vi "PH_PILS.vis ResetEOKnob.vi"(0 "i ref in":refnum<vi>, 5 "error IO":errorcluster) -> (14 "i ref out":refnum<vi>, 19 "error out":errorcluster)   [LabVIEW 2014, in "PH_PILS.lvlib"]
uses:
  PH_PILS.lvlib
  PH_Basics/PH_SystemInformation/PH_SystemInformation.lvlib
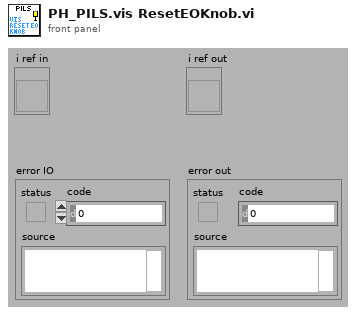
[diagram p1: front panel]
types:
  T1 = typedef "PH_PILS.lvlib/PH_PILS.i attribute.ctl" = cluster{"Boolean":cluster{"GUI Ref":refnum<vi>, "Status":i32}[], "GUI Refs Exp. Shutters":cluster{"1":refnum<vi>, "2":refnum<vi>, "3":refnum<vi>, "4":refnum<vi>}, "Tristate2Run GUI Refs":refnum<vi>[], "EO-Likes":cluster{"GUI Ref":refnum<vi>, "Status":i32}[], "Operation Mode":cluster{"Operation Mode":T2, "GUI":cluster{"Ref State":refnum<vi>, "Ref":refnum<vi>}, "Servicemode":cluster{"Tagname":string, "Status":i32}, "Labormode":cluster{"Tagname":string, "Status":i32}, "Searchmode":cluster{"Tagname":string, "Status":i32}, "Shotmode":cluster{"Tagname":string, "Status":i32}}, "Submode":cluster{"Submode":T3, "GUI":cluster{"Ref State":refnum<vi>, "Ref":refnum<vi>}, "Submode":cluster{"Tagname":string, "Status":i32}}, "Experiment":cluster{"Experiment":enum16{"unknown", "intern", "4 (Z6)", "3", "2", "1"}, "GUI":cluster{"Ref State":refnum<vi>, "Ref":refnum<vi>}, "intern":cluster{"Tagname":string, "Status":i32}, "Exp 4":cluster{"Tagname":string, "Status":i32}, "Exp 3":cluster{"Tagname":string, "Status":i32}, "Exp 2":cluster{"Tagname":string, "Status":i32}, "Exp 1":cluster{"Tagname":string, "Status":i32}}, "TristateNormal":cluster{"GUI Ref":refnum<vi>, "Status":i32}[], "Door Tags":cluster{"GUI Ref":refnum<vi>, "Status":i32}[], "GUIlessTags":cluster{"Name":string, "Status":i32}[], "Beamline GUI Refs":refnum<vi>[], "Special Boolean":cluster{"GUI Ref":refnum<vi>, "Status":i32}[], "Laserpower":cluster{"GUI Ref":refnum<vi>, "Status":i32}[], "Shutter":cluster{"GUI Ref":refnum<vi>, "Status":i32}[], "Tristate EO Like":cluster{"GUI Ref":refnum<vi>, "Status":i32}[], "PP":cluster{"GUI Ref":refnum<vi>, "Status":i32, "Head Ref":refnum<vi>, "Slider Ref":refnum<vi>}[], "Switch Knobs":cluster{"GUI Ref":refnum<vi>, "Status":i32}[], "Latch Knob GUI Refs":refnum<vi>[], "FailureCounter":i32, "Enabled Status":cluster{"Laser":i32, "PreAmp":i32, "MainAmp":i32}, "Mercury":refnum<vi>, "Instance Rods":string, "Logfile":path, "Beckhoff-Instance Internal":string, "Beckhoff-Instance External":string, "Enabling Rights":cluster{"Name":string, "Password":string, "PA?":bool, "MA?":bool, "Exp?":bool}[]}
  T2 = typedef "PH_PILS.lvlib/PH_PILS.Operation Mode.ctl" = enum16{"unknown", "Service", "Labor", "Search", "Shot"}
  T3 = typedef "PH_PILS.lvlib/PH_PILS.Submode.ctl" = enum16{"unknown", "HV-Normal", "HV-Test"}
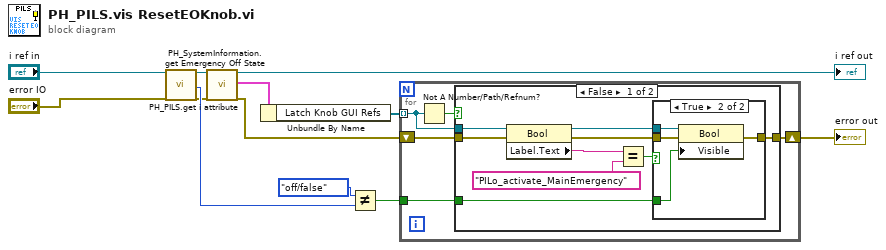
[diagram p0: block diagram]
diagram:
  n1 = call "PH_SystemInformation.get Emergency Off State.vi"("i ref in"="i ref in", "error in (no error)"="error IO") -> ("i ref out"=w1:refnum<vi>, "Emergency Off State"=w7:enum16{"no info", "off/false", "Alarm"}, "error out"=w3:errorcluster)  [unwired: 15 in]
  n2 = call "PH_PILS.get i attribute.vi"("i ref in"=w1, "error in (no error)"=w3) -> ("i ref out"=→"i ref out":refnum<vi>, "i attribute"=w11:T1, "error out"=w5:errorcluster)  [unwired: 15 in]
  n3 = Unbundle By Name(w11) -> ("Latch Knob GUI Refs"=w9:refnum<vi>[])
  n4 = Not Equal?(x=enum16{"no info", "off/false", "Alarm"}."off/false", y=w7) -> (x != y?=w8:bool)
  n5 = for {
    tunnel: w8 -> [w15]
    shift-right: [w16] -> w10
    shift-left: w5 -> [w14]
    tunnel: w9 -> [w13] mode=indexing
    n6 = Not A Number/Path/Refnum?(number/path/refnum=w13) -> (NaN/Path/Refnum?=w17:bool)
    n7 = case shown="False" w17 {
      tunnel: w14 -> [w24 w32]
      tunnel: w13 -> [w22 _]
      tunnel: [w26 w32] -> w16
      tunnel: w15 -> [w25 _]
      frame False {
        n8 = property class="Bool"(reference=w22, error in=w24) -> (reference out=w21:refnum<vi>, error out=w23:errorcluster, "Label.Text"=w20:string)
        n9 = Equal?(x=w20, y="PILo_activate_MainEmergency") -> (x = y?=w18:bool)
        n10 = case shown="True" w18 {
          tunnel: [w27 w31] -> w26
          tunnel: w25 -> [_ w30]
          tunnel: w23 -> [w27 w29]
          tunnel: w21 -> [_ w28]
          frame False {
          }
          frame True {
            n11 = property class="Bool"(reference=w28, error in=w29, "Visible"=w30) -> (error out=w31:errorcluster)  [unwired: 1 out]
          }
        }
      }
      frame True {
      }
    }
  }
  "error out" <- w10
